vi "Finalize.vi"(8 "error in":errorcluster, 11 "Plugin in":refnum<class "Digital Output Handler.lvclass">) -> (0 "error out":errorcluster, 3 "Plugin out":refnum<class "Digital Output Handler.lvclass">)   [LabVIEW 2023, in "Digital Output Handler.lvlib" / "Digital Output Handler.lvclass"]
uses:
  Digital Output Handler.lvclass
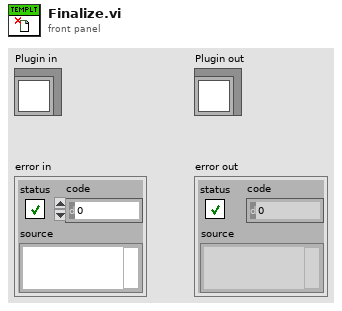
[diagram p1: front panel]
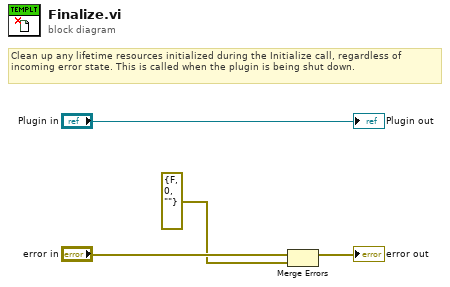
[diagram p0: block diagram]
diagram:
  # "Clean up any lifetime resources initialized during the Initialize call, regardless of incoming error state. This is called when the plugin is being shut down."
  n1 = Merge Errors("error in", errorcluster {"status"=FALSE, "code"=0, "source"=""} ("error in")) -> (→"error out":errorcluster)
  "Plugin out" <- "Plugin in"
